vi "Waveform data class VI - add waveform data.vi"(0 "Waveform data in":refnum<class "Waveform data.lvclass">, 5 "angle":dbl, 7 "displacement":dbl, 11 "error in (no error)":errorcluster) -> (4 "Waveform data out":refnum<class "Waveform data.lvclass">, 15 "error out":errorcluster)   [LabVIEW 2010, in "Waveform data.lvclass"]
uses:
  Waveform data.lvclass
  Waveform data.lvclass/Waveform data.ctl
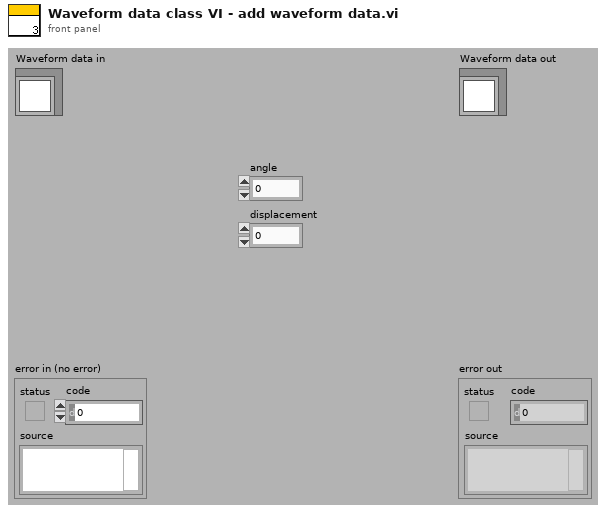
[diagram p1: front panel]
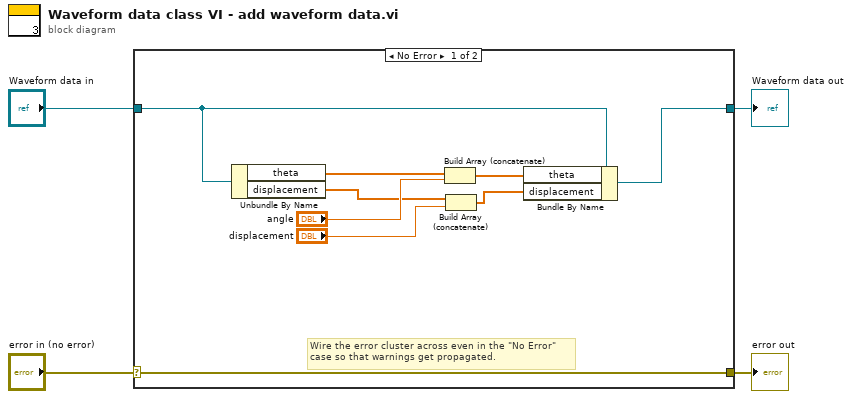
[diagram p0: block diagram]
diagram:
  n1 = case shown="No Error" "error in (no error)" {
    selector: "error in (no error)" -> [w13 w15]
    tunnel: [w13 w15] -> w3
    tunnel: [w7 w14] -> w1
    tunnel: "Waveform data in" -> [w8 w14]
    frame No Error {
      # "Wire the error cluster across even in the \"No Error\"\ncase so that warnings get propagated."
      n2 = Unbundle By Name(w8) -> ("theta"=w10:dbl[], "displacement"=w9:dbl[])
      n3 = Build Array (concatenate)(w10, "angle") -> (w6:dbl[])
      n4 = Build Array (concatenate)(w9, "displacement") -> (w5:dbl[])
      n5 = Bundle By Name(cluster=w8, "theta"=w6, "displacement"=w5) -> (w7:refnum<class "Waveform data.lvclass">)
    }
    frame Error {
    }
  }
  "error out" <- w3
  "Waveform data out" <- w1
